vi "Webcam Face detect.vi"() -> ()   [LabVIEW 2014]
uses:
  <vilib>/vision/NI_Vision_Development_Module.lvlib
  <vilib>/vision/driver/NI_Vision_Acquisition_Software.lvlib
panel:
  out "error out":errorcluster
  in  "Rotation Angle Ranges (degrees)":cluster{sgl, sgl}[](array[cluster])
  out "Matches[0]":T1
  in  "Minimum Match Score":sgl=800.0 min=0 max=1000 format="%.2f"
  out "error out 2":errorcluster
  out "x-y":u32
  in  "milliseconds to wait":u32
  in  "error in (no error)":errorcluster
  in  "stop":bool
  out "Image":T2(plugin-control)
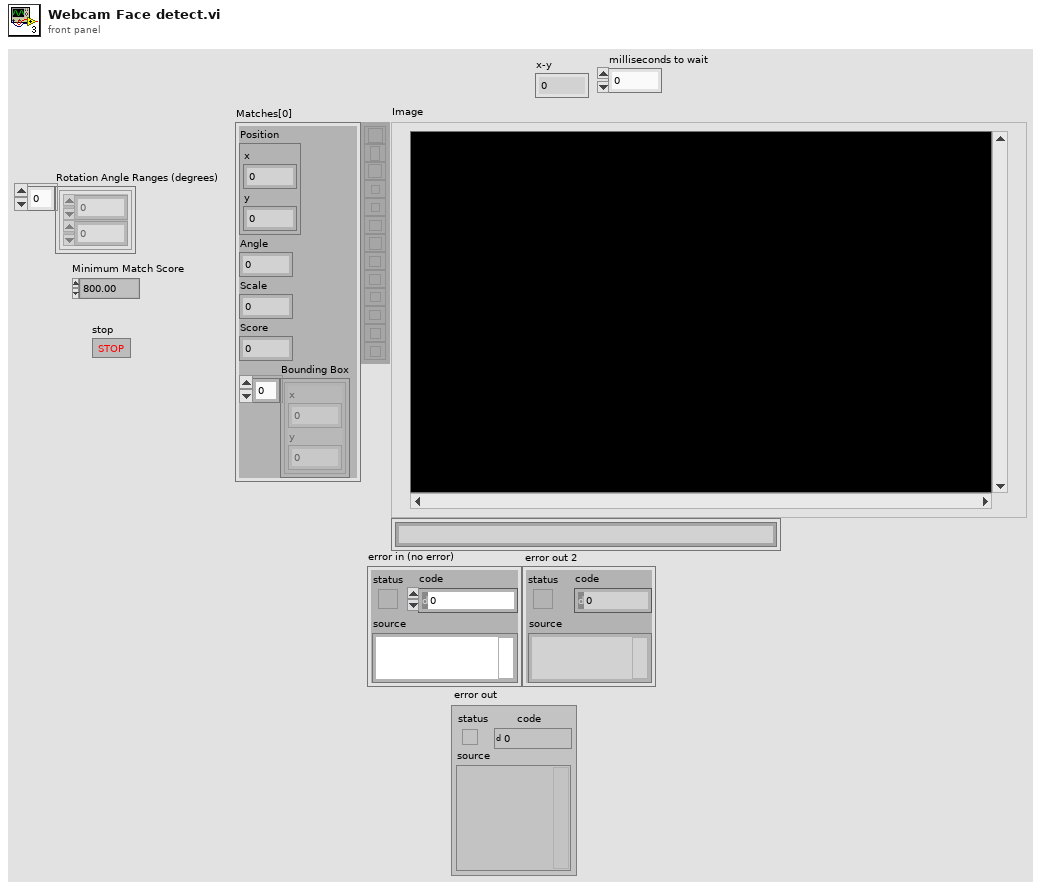
[diagram p1: front panel]
types:
  T1 = cluster{"Position":cluster{"x":sgl, "y":sgl}, "Angle":sgl, "Scale":sgl, "Score":sgl, "Bounding Box":cluster{"x":sgl, "y":sgl}[]}
  T2 = typedef "IMAQ Image.ctl" = refnum<image>
  T3 = typedef "IMAQdx.ctl" = refnum<k21>
  T4 = typedef "IMAQ Rectangle" = cluster{"Left":i32, "Top":i32, "Right":i32, "Bottom":i32, "Rotation":dbl}
  T5 = cluster{"Position":cluster{"x":sgl, "y":sgl}, "Angle":sgl, "Scale":sgl, "Score":sgl, "Bounding Box":cluster{"x":sgl, "y":sgl}[]}[]
  T6 = cluster{"Matches[0]":cluster{"Position":cluster{"x":sgl, "y":sgl}, "Angle":sgl, "Scale":sgl, "Score":sgl, "Bounding Box":cluster{"x":sgl, "y":sgl}[]}, "Matches[1]":cluster{"Position":cluster{"x":sgl, "y":sgl}, "Angle":sgl, "Scale":sgl, "Score":sgl, "Bounding Box":cluster{"x":sgl, "y":sgl}[]}, "Matches[2]":cluster{"Position":cluster{"x":sgl, "y":sgl}, "Angle":sgl, "Scale":sgl, "Score":sgl, "Bounding Box":cluster{"x":sgl, "y":sgl}[]}, "Matches[3]":cluster{"Position":cluster{"x":sgl, "y":sgl}, "Angle":sgl, "Scale":sgl, "Score":sgl, "Bounding Box":cluster{"x":sgl, "y":sgl}[]}, "Matches[4]":cluster{"Position":cluster{"x":sgl, "y":sgl}, "Angle":sgl, "Scale":sgl, "Score":sgl, "Bounding Box":cluster{"x":sgl, "y":sgl}[]}, "Matches[5]":cluster{"Position":cluster{"x":sgl, "y":sgl}, "Angle":sgl, "Scale":sgl, "Score":sgl, "Bounding Box":cluster{"x":sgl, "y":sgl}[]}, "Matches[6]":cluster{"Position":cluster{"x":sgl, "y":sgl}, "Angle":sgl, "Scale":sgl, "Score":sgl, "Bounding Box":cluster{"x":sgl, "y":sgl}[]}, "Matches[7]":cluster{"Position":cluster{"x":sgl, "y":sgl}, "Angle":sgl, "Scale":sgl, "Score":sgl, "Bounding Box":cluster{"x":sgl, "y":sgl}[]}, "Matches[8]":cluster{"Position":cluster{"x":sgl, "y":sgl}, "Angle":sgl, "Scale":sgl, "Score":sgl, "Bounding Box":cluster{"x":sgl, "y":sgl}[]}}
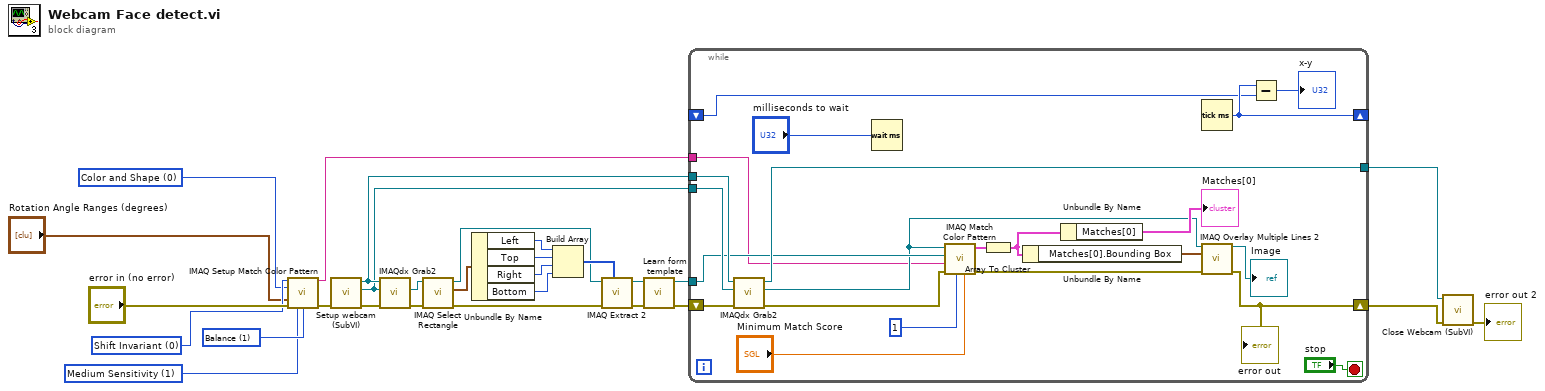
[diagram p0: block diagram]
diagram:
  w21 = u32 1 items=["Low Sensitivity", "Medium Sensitivity", "High Sensitivity"] ("Color Sensitivity")
  w22 = u32 1 items=["Conservative", "Balance", "Aggressive", "Very Aggressive"] ("Search Strategy")
  w24 = u32 0 items=["Color and Shape", "Color", "Shape"] ("Match Feature Mode")
  w25 = u32 0 items=["Shift Invariant", "Rotation Invariant"] ("Match Mode")
  n1 = call "IMAQ Setup Match Color Pattern"("Match Mode"=w25, "Match Feature Mode"=w24, "Rotation Angle Ranges (degrees)"="Rotation Angle Ranges (degrees)", "error in (no error)"="error in (no error)", "Color Sensitivity"=w21, "Search Strategy"=w22) -> ("Match Color Pattern Setup Data"=w4:string, "error out"=w3:errorcluster)  [unwired: 8 in]
  n2 = call "Setup webcam (SubVI).vi"("error in (no error)"=w3) -> ("error out"=w2:errorcluster, "New Image"=w7:T2, "Refnum out"=w8:T3)  [unwired: 8 in]
  n3 = call <vilib>:"IMAQdx Grab2.vi"("error in"=w2, "Image In"=w7, "Session In"=w8) -> ("error out"=w19:errorcluster, "Image Out"=w20:T2)  [unwired: 5 in, 2 out]
  n4 = call "IMAQ Select Rectangle"("error in (no error)"=w19, "Image In"=w20) -> ("error out"=w11:errorcluster, "Rectangle"=w18:T4, "Image Out (duplicate)"=w12:T2)  [unwired: 6 in, 1 out]
  n5 = Unbundle By Name(w18) -> ("Left"=w17:i32, "Top"=w16:i32, "Right"=w15:i32, "Bottom"=w14:i32)
  n6 = Build Array(w17, w16, w15, w14) -> (w13:i32[])
  n7 = call "IMAQ Extract 2"("Optional Rectangle"=w13, "error in (no error)"=w11, "Image Src"=w12) -> ("error out"=w10:errorcluster, "Image Dst Out"=w6:T2)  [unwired: 7 in]
  n8 = call "Learn form template.vi"("error in (no error)"=w10, "Template Image"=w6) -> ("error out"=w9:errorcluster, "Refnum out"=w5:T2)  [unwired: 8 in]
  n9 = while {
    tunnel: w5 -> [w31]
    shift-right: [w44] -> _
    shift-left: _ -> [w43]
    tunnel: w8 -> [w41]
    tunnel: w7 -> [w40]
    tunnel: [w33] -> w27
    tunnel: w4 -> [w29]
    shift-right: [w48] -> w1
    shift-left: w9 -> [w34]
    stop <- "stop" stop-if-true
    n10 = call <vilib>:"IMAQdx Grab2.vi"("error in"=w34, "Image In"=w40, "Session In"=w41) -> ("error out"=w32:errorcluster, "Image Out"=w30:T2, "Session Out"=w33:T3)  [unwired: 5 in, 1 out]
    n11 = Wait (ms)(milliseconds to wait="milliseconds to wait") -> ()  [unwired: 1 out]
    n12 = call "IMAQ Match Color Pattern"("Minimum Match Score"="Minimum Match Score", "Number of Matches Requested"=1, "error in (no error)"=w32, "Match Color Pattern Setup Data"=w29, "Template Image"=w31, "Image"=w30) -> ("error out"=w39:errorcluster, "Matches"=w47:T5)  [unwired: 3 in, 1 out]
    n13 = Array To Cluster(array=w47) -> (cluster=w36:T6)
    n14 = Unbundle By Name(w36) -> ("Matches[0].Bounding Box"=w50:cluster{"x":sgl, "y":sgl}[])
    n15 = Unbundle By Name(w36) -> ("Matches[0]"=→"Matches[0]":T1)
    n16 = Tick Count (ms)() -> (millisecond timer value=w44:u32)
    n17 = call "IMAQ Overlay Multiple Lines 2"("Image"=w30, "Line End Points"=w50, "error in (no error)"=w39) -> ("Image Out"=→"Image":T2, "error out"=w48:errorcluster)  [unwired: 11 in]
    "error out" <- w48
    n18 = Subtract(x=w44, y=w43) -> (x-y=→"x-y":u32)
  }
  n19 = call "Close Webcam (SubVI).vi"("error in (no error)"=w1, "Refnum in"=w27) -> ("error out"=→"error out 2":errorcluster)  [unwired: 9 in]
